vi "Banco2 da Banco3.vi"() -> ()   [LabVIEW 2019]
panel:
  out "gestisci linea banco2?":bool
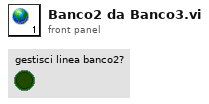
[diagram p1: front panel]
diagram:
